vi "Multi_Auto-Correlation.vi"(7 "Velocity arrays":dbl[][](array[numeric]) format="%.2f") -> (3 "Auto-Corr":dbl[][](array[numeric]) format="%.2f")   [LabVIEW 2010]
uses:
  Globals/Meas_global.vi
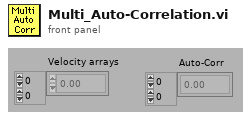
[diagram p1: front panel]
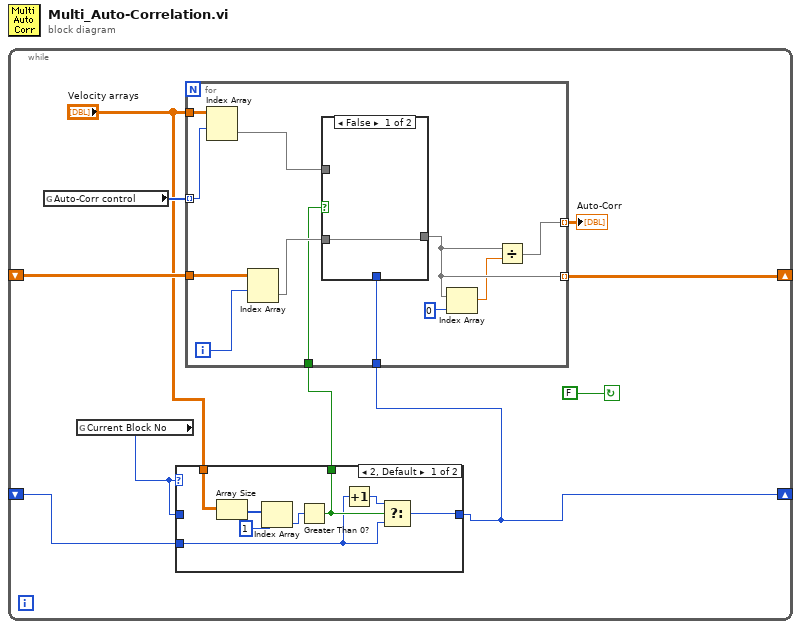
[diagram p0: block diagram]
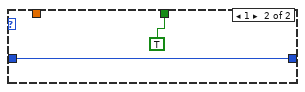
[diagram p2: hidden frame]
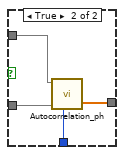
[diagram p3: hidden frame]
diagram:
  n1 = while {
    shift-left: _ -> [w7]
    shift-right: [w9] -> _
    shift-right: [w1] -> _
    shift-left: _ -> [w4]
    stop <- FALSE continue-if-true
    n2 = global read "Meas_global.vi" "Auto-Corr control"() -> (w8:i32[])
    n3 = global read "Meas_global.vi" "Current Block No"() -> (w5:i32)
    n4 = case shown="2, Default" w5 {
      tunnel: [w11 w20] -> w1
      tunnel: w5 -> [_ w20]
      tunnel: "Velocity arrays" -> [w18 _]
      tunnel: [w14 TRUE] -> w2
      tunnel: w4 -> [w12 _]
      frame 2, Default {
        n5 = Array Size(array=w18) -> (size(s)=w17:i32[])
        n6 = Index Array(array=w17, index=1) -> (element=w15:i32)
        n7 = Greater Than 0?(x=w15) -> (x > 0?=w14:bool)
        n8 = Increment(x=w12) -> (x+1=w13:i32)
        n9 = Select(t=w13, s=w14, f=w12) -> (s? t:f=w11:i32)
      }
      frame 1 {
      }
    }
    n10 = for {
      tunnel: w8 -> [w30] mode=indexing
      tunnel: "Velocity arrays" -> [w32]
      tunnel: [w25] -> w10 mode=indexing
      tunnel: [w24] -> w9 mode=indexing
      tunnel: w7 -> [w27]
      tunnel: w2 -> [w22]
      tunnel: w1 -> [w21]
      i -> [w29]
      n11 = Index Array(array=w32, index (row)=w30) -> (element=w31:dbl[])  [unwired: 1 in]
      n12 = Index Array(array=w27, index (row)=w29) -> (element=w28:dbl[])  [unwired: 1 in]
      n13 = case shown="False" w22 {
        tunnel: w31 -> [_ w37]
        tunnel: w28 -> [w33 w36]
        tunnel: [w33 w35] -> w24
        tunnel: w21 -> [_ w34]
        frame False {
        }
        frame True {
          n14 = call "Autocorrelation_ph.vi"("X"=w37, "Autocorrelation of X"=w36, "Block No"=w34) -> ("Autocorrelation of X"=w35:dbl[])  [unwired: 2 in, 1 out]
        }
      }
      n15 = Index Array(array=w24, index=0 ("Index")) -> (element=w23:dbl)
      n16 = Divide(x=w24, y=w23) -> (x/y=w25:dbl[])
    }
    "Auto-Corr" <- w10
  }
